vi "libssh2_knownhost_readfile - valid file - returns number of hosts.vi"() -> ()   [LabVIEW 2017, in "unit_tests.lvlib"]
uses:
  unit_tests.lvlib
  libssh2/libssh2_init_default.vi
  libssh2/libssh2_session_init_ex.vi
  libssh2/libssh2.lvlib
  <vilib>/PNR/Transparent Assertions/Transparent Assertions/Transparent Assertions.lvlib
panel:
  out "error out":errorcluster
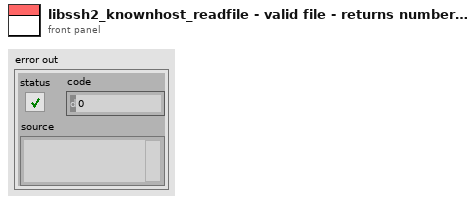
[diagram p1: front panel]
types:
  T1 = typedef "libssh2.lvlib/Session Refnum.ctl" = refnum<k1>
  T2 = typedef "libssh2.lvlib/Host Key Database Refnum.ctl" = refnum<k1>
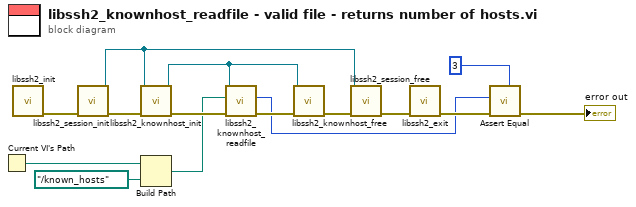
[diagram p0: block diagram]
diagram:
  n1 = Current VI's Path() -> (path=w3:path)
  n2 = call-poly "libssh2_init.vi"() -> ("error out"=w14:errorcluster)  [unwired: 11 in]
  n3 = call "libssh2_session_init.vi"("error in (no error)"=w14) -> ("error out"=w13:errorcluster, "session"=w10:T1)  [unwired: 9 in]
  n4 = call "libssh2_knownhost_init.vi"("error in (no error)"=w13, "session"=w10) -> ("error out"=w8:errorcluster, "host key database"=w6:T2)  [unwired: 8 in]
  n5 = Build Path(base path=w3, name or relative path=path "../known_hosts" ("filename")) -> (appended path=w1:path)
  n6 = call "libssh2_knownhost_readfile.vi"("error in (no error)"=w8, "filename"=w1, "host key database"=w6) -> ("error out"=w7:errorcluster, "hosts added"=w5:i32)  [unwired: 7 in]
  n7 = call "libssh2_knownhost_free.vi"("error in (no error)"=w7, "host key database"=w6) -> ("error out"=w9:errorcluster)  [unwired: 9 in]
  n8 = call "libssh2_session_free.vi"("error in (no error)"=w9, "session"=w10) -> ("error out"=w12:errorcluster)  [unwired: 9 in]
  n9 = call "libssh2_exit.vi"("error in (no error)"=w12) -> ("error out"=w11:errorcluster)  [unwired: 10 in]
  n10 = call <vilib>:"Assert Equal.vi"("Expected"=3 ("hosts added"), "error in (no error)"=w11, "Actual"=w5) -> ("error out"=→"error out":errorcluster)  [unwired: 8 in]
